vi "ENVIODEANGULOS.vi"(0 "dato A":i32, 1 "dato B":i32, 2 "dato C":i32, 3 "dato D":i32, 4 "dato E":i32, 5 "fin de cadena":string=" S") -> (19 "cadena a enviar":string)   [LabVIEW 2017]
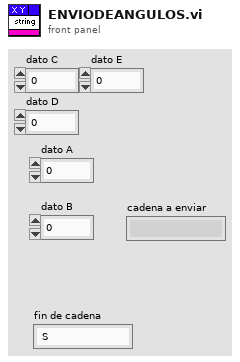
[diagram p1: front panel]
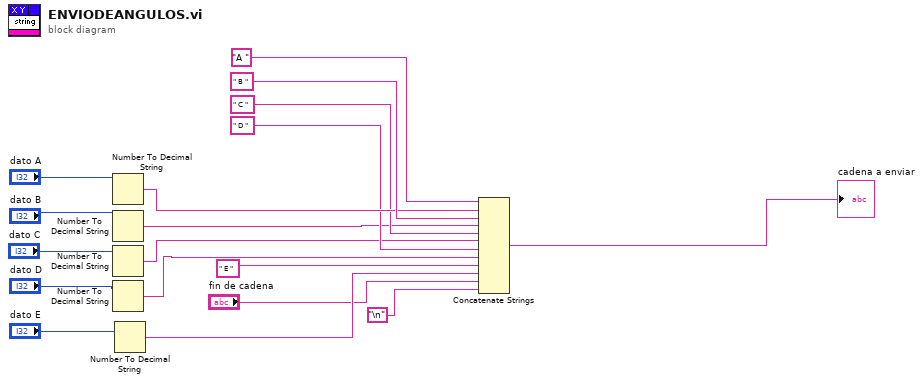
[diagram p0: block diagram]
diagram:
  n1 = Number To Decimal String(number="dato A") -> (decimal integer string=w16:string)  [unwired: 1 in]
  n2 = Number To Decimal String(number="dato B") -> (decimal integer string=w10:string)  [unwired: 1 in]
  n3 = Number To Decimal String(number="dato C") -> (decimal integer string=w9:string)  [unwired: 1 in]
  n4 = Number To Decimal String(number="dato D") -> (decimal integer string=w8:string)  [unwired: 1 in]
  n5 = Number To Decimal String(number="dato E") -> (decimal integer string=w4:string)  [unwired: 1 in]
  n6 = Concatenate Strings("A " ("string"), w16, " B " ("string"), w10, " C " ("string"), w9, " D " ("string"), w8, " E " ("string"), w4, "fin de cadena", "\n") -> (→"cadena a enviar":string)
